vi "Match Camera.vi"(8 "error in (no error)":errorcluster, 10 "IMAQdx Data":T1 {"SerialNumberHigh" format="%x"; "SerialNumberLow" format="%x"}, 11 "FlexWorktable in":refnum<class "FlexWorktable.lvclass">) -> (0 "error out":errorcluster, 1 "Camera Matched":bool, 2 "Matched Camera Name":string, 3 "FlexWorktable out":refnum<class "FlexWorktable.lvclass">)   [LabVIEW 2017, in "FlexWorktable.lvclass"]
uses:
  FlexWorktable.lvclass
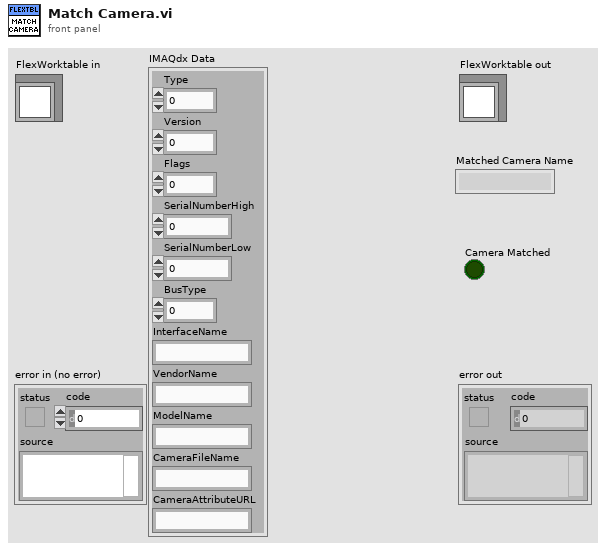
[diagram p1: front panel]
types:
  T1 = cluster{"Type":u32, "Version":u32, "Flags":u32, "SerialNumberHigh":u32, "SerialNumberLow":u32, "BusType":u32, "InterfaceName":string, "VendorName":string, "ModelName":string, "CameraFileName":string, "CameraAttributeURL":string}
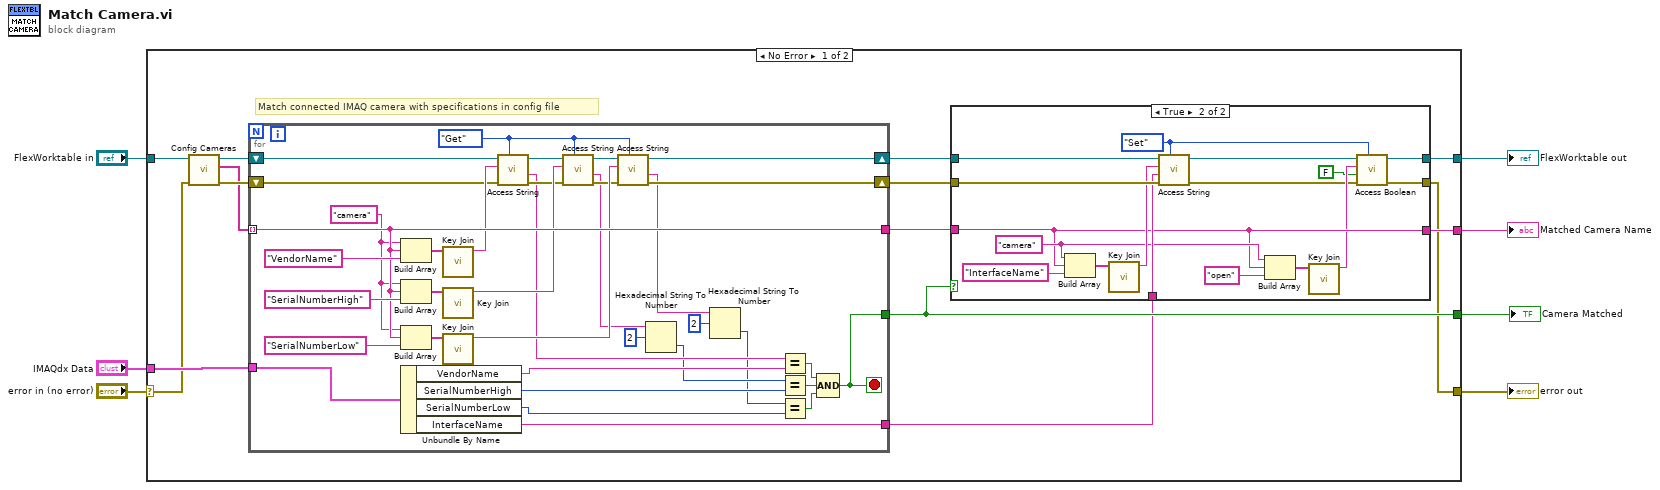
[diagram p0: block diagram]
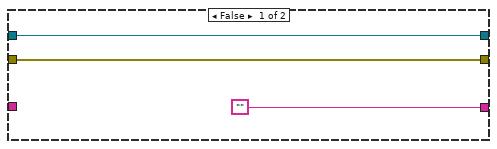
[diagram p2: hidden frame]
diagram:
  n1 = case shown="No Error" "error in (no error)" {
    selector: "error in (no error)" -> [w19 w79]
    tunnel: "IMAQdx Data" -> [w21 _]
    tunnel: [w12 w78] -> w6
    tunnel: [w8 w79] -> w4
    tunnel: "FlexWorktable in" -> [w20 w78]
    tunnel: [w10 _] -> w2
    tunnel: [w15 _] -> w1
    frame No Error {
      # "Match connected IMAQ camera with specifications in config file"
      n2 = call "Config Cameras.vi"("error in (no error)"=w19, "FlexWorktable in"=w20) -> ("error out"=w17:errorcluster, "Array"=w16:string[], "FlexWorktable out"=w18:refnum<class "FlexWorktable.lvclass">)  [unwired: 7 in]
      n3 = for {
        tunnel: w16 -> [w65] mode=indexing
        tunnel: w21 -> [w77]
        tunnel: [w72] -> w15
        tunnel: [w65] -> w11
        shift-right: [w52] -> w14
        shift-left: w18 -> [w60]
        shift-right: [w49] -> w13
        shift-left: w17 -> [w50]
        tunnel: [w48] -> w9
        stop <- w72 stop-if-true
        w51 = enum16{"Get", "Set"}."Get" ("Get/Set")
        w64 = "camera"
        n4 = Build Array(w64, w65, "VendorName" ("key")) -> (w69:string[])
        n5 = Build Array(w64, w65, "SerialNumberHigh" ("key")) -> (w62:string[])
        n6 = Build Array(w64, w65, "SerialNumberLow" ("key")) -> (w63:string[])
        n7 = Unbundle By Name(w77) -> ("VendorName"=w76:string, "SerialNumberHigh"=w70:u32, "SerialNumberLow"=w71:u32, "InterfaceName"=w48:string)
        n8 = call "Key Join.vi"("Key Elements"=w69) -> ("Key"=w61:string)  [unwired: 10 in]
        n9 = call "Key Join.vi"("Key Elements"=w62) -> ("Key"=w59:string)  [unwired: 10 in]
        n10 = call "Key Join.vi"("Key Elements"=w63) -> ("Key"=w56:string)  [unwired: 10 in]
        n11 = call-dynamic "Access String.vi"("Get/Set"=w51, "error in (no error)"=w50, "Key"=w61, "FlexWorktable in"=w60) -> ("error out"=w55:errorcluster, "Value out"=w53:string, "FlexWorktable out"=w58:refnum<class "FlexWorktable.lvclass">)  [unwired: 5 in]
        n12 = call-dynamic "Access String.vi"("Get/Set"=w51, "error in (no error)"=w55, "Key"=w59, "FlexWorktable in"=w58) -> ("error out"=w54:errorcluster, "Value out"=w47:string, "FlexWorktable out"=w57:refnum<class "FlexWorktable.lvclass">)  [unwired: 5 in]
        n13 = call-dynamic "Access String.vi"("Get/Set"=w51, "error in (no error)"=w54, "Key"=w56, "FlexWorktable in"=w57) -> ("error out"=w49:errorcluster, "Value out"=w43:string, "FlexWorktable out"=w52:refnum<class "FlexWorktable.lvclass">)  [unwired: 5 in]
        n14 = Hexadecimal String To Number(string=w47, offset=2) -> (number=w46:u32)  [unwired: 1 in, 1 out]
        n15 = Hexadecimal String To Number(string=w43, offset=2) -> (number=w42:u32)  [unwired: 1 in, 1 out]
        n16 = Equal?(x=w53, y=w76) -> (x = y?=w75:bool)
        n17 = Equal?(x=w46, y=w70) -> (x = y?=w74:bool)
        n18 = Equal?(x=w42, y=w71) -> (x = y?=w73:bool)
        n19 = Compound Arithmetic op=AND(w75, w74, w73) -> (w72:bool)
      }
      n20 = case shown="True" w15 {
        tunnel: w14 -> [w24 w41]
        tunnel: w13 -> [w23 w40]
        tunnel: [w24 w30] -> w12
        tunnel: [w23 w25] -> w8
        tunnel: w11 -> [_ w33]
        tunnel: ["" w33] -> w10
        tunnel: w9 -> [_ w39]
        frame False {
        }
        frame True {
          w34 = "camera"
          w27 = enum16{"Get", "Set"}."Set" ("Get/Set")
          n21 = Build Array(w34, w33, "InterfaceName") -> (w38:string[])
          n22 = call "Key Join.vi"("Key Elements"=w38) -> ("Key"=w37:string)  [unwired: 10 in]
          n23 = call-dynamic "Access String.vi"("Get/Set"=w27, "error in (no error)"=w40, "Value in"=w39, "Key"=w37, "FlexWorktable in"=w41) -> ("error out"=w28:errorcluster, "FlexWorktable out"=w31:refnum<class "FlexWorktable.lvclass">)  [unwired: 4 in, 1 out]
          n24 = Build Array(w34, w33, "open" ("element")) -> (w35:string[])
          n25 = call "Key Join.vi"("Key Elements"=w35) -> ("Key"=w29:string)  [unwired: 10 in]
          n26 = call-dynamic "Access Boolean.vi"("Get/Set"=w27, "error in (no error)"=w28, "Value in"=FALSE, "Key"=w29, "FlexWorktable in"=w31) -> ("error out"=w25:errorcluster, "FlexWorktable out"=w30:refnum<class "FlexWorktable.lvclass">)  [unwired: 4 in, 1 out]
        }
      }
    }
    frame Error {
    }
  }
  "error out" <- w4
  "FlexWorktable out" <- w6
  "Matched Camera Name" <- w2
  "Camera Matched" <- w1
